vi "manual graph pascal triangle curve.vi"() -> ()   [LabVIEW 2009]
panel:
  in  "milliseconds to wait":u32(slide) scale=1.0..1000.0
  in  "stop":bool
  out "Waveform Graph":dbl[](graph)
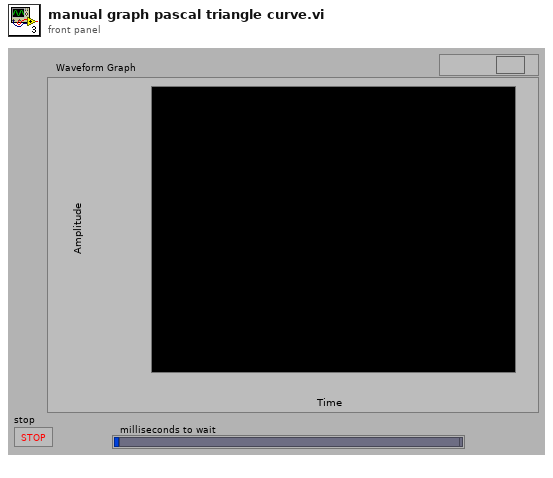
[diagram p1: front panel]
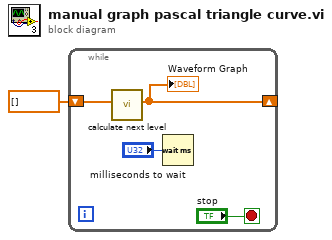
[diagram p0: block diagram]
diagram:
  n1 = while {
    shift-right: [w5] -> _
    shift-left: dbl[] [] ("next level") -> [w4]
    stop <- "stop" stop-if-true
    n2 = call "calculate next level.vi"("pascal's triangle"=w4) -> ("next level"=w5:dbl[])  [unwired: 10 in]
    "Waveform Graph" <- w5
    n3 = Wait (ms)(milliseconds to wait="milliseconds to wait") -> ()  [unwired: 1 out]
  }
